vi "connect.vi"(8 "error in (no error)":errorcluster, 11 "MyComics.org_class in":refnum<class "MyComics.org_class.lvclass">) -> (0 "error out":errorcluster, 3 "MyComics.org_class out":refnum<class "MyComics.org_class.lvclass">)   [LabVIEW 2024, in "MyComics.org_class.lvclass"]
uses:
  MyComics.org_class.lvclass
  MyComics.org_class.lvclass/MyComics.org_class.ctl
  <vilib>/httpClient/LabVIEWHTTPClient.lvlib
  <vilib>/httpClient/POSTBuffer.vi
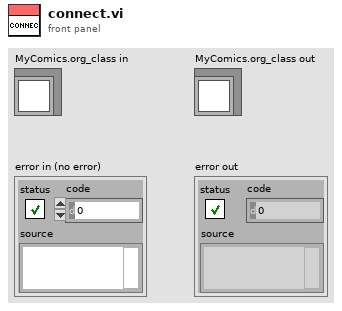
[diagram p1: front panel]
types:
  T1 = typedef "LabVIEWHTTPClient.lvlib/ClientHandle.ctl" = refnum<k1>
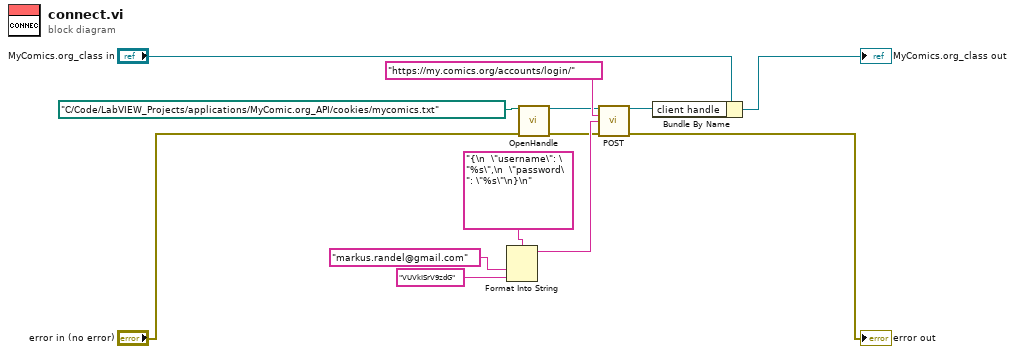
[diagram p0: block diagram]
diagram:
  n1 = Format Into String(format string="{\n  \"username\": \"%s\",\n  \"password\": \"%s\"\n}\n", "markus.randel@gmail.com", "VUVkISrV9zdG") -> (resulting string=w9:string)  [unwired: 2 in, 1 out]
  n2 = call <vilib>:"OpenHandle.vi"("cookie file"=path "C:/Code/LabVIEW_Projects/applications/MyComic.org_API/cookies/mycomics.txt", "error in (no error)"="error in (no error)") -> ("client handle out"=w7:T1, "error out"=w6:errorcluster)  [unwired: 12 in]
  n3 = call-poly <vilib>:"POST.vi"("client handle"=w7, "url"="https://my.comics.org/accounts/login/", "buffer"=w9, "error in (no error)"=w6) -> ("client handle out"=w5:T1, "error out"=→"error out":errorcluster)  [unwired: 8 in, 2 out]
  n4 = Bundle By Name(cluster="MyComics.org_class in", "client handle"=w5) -> (→"MyComics.org_class out":refnum<class "MyComics.org_class.lvclass">)
